vi "Exercise 6.1 PID Host GUI DataLog.vi"() -> ()   [LabVIEW 2014]
doc: "This example demonstrates how to implement a STM client which receives messages from the server.\n\nThe server needs to be started before the client."
uses:
  <vilib>/NI/STM/compatibility/STM Read Meta Data (TCP Ref).vi
  <vilib>/NI/STM/compatibility/STM Read Message (TCP).vi
  <vilib>/Utility/file.llb/Write To Spreadsheet File (DBL).vi
  <vilib>/Utility/file.llb/Write To Spreadsheet File (string).vi
  <vilib>/NI/STM/compatibility/STM Get Connection Reference (TCP).vi
  <vilib>/wsapi/NI_WebServices.lvlib
  <vilib>/Platform/browser.llb/Open URL in Default Browser (string).vi
panel:
  out "Output (MV)":dbl(graph)
  out "HL":bool
  out "LL":bool
  out "Max":dbl
  out "Min":dbl
  out "SP":dbl(knob) scale=0.0..100.0
  out "PV":dbl(knob) scale=0.0..100.0
  out "Monitor Chart":T1(graph)
  in  "Target IP Address":string="192.168.5.1"
  in  "stop":bool
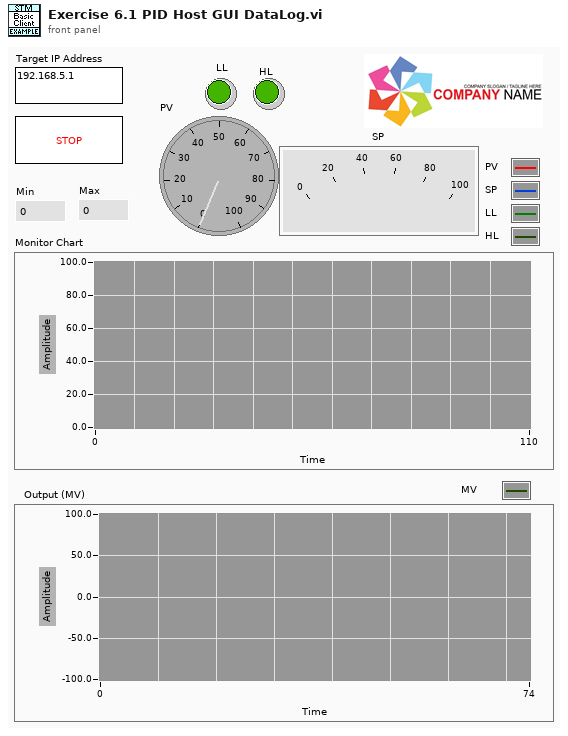
[diagram p1: front panel]
types:
  T1 = cluster{"PV":dbl, "SP":dbl, "Min":dbl, "Max":dbl}
  T2 = typedef "stm_TCP Connection Info.ctl" = cluster{"connection ID":refnum<k5>, "Meta data":T3[]}
  T3 = typedef "stm_MetaDataElement.ctl" = string
  T4 = typedef "imagedata.ctl" = cluster{"image type":i32, "image depth":i32, "image":u8[], "mask":u8[], "colors":u32[], "Rectangle":cluster{"left":i16, "top":i16, "right":i16, "bottom":i16}}
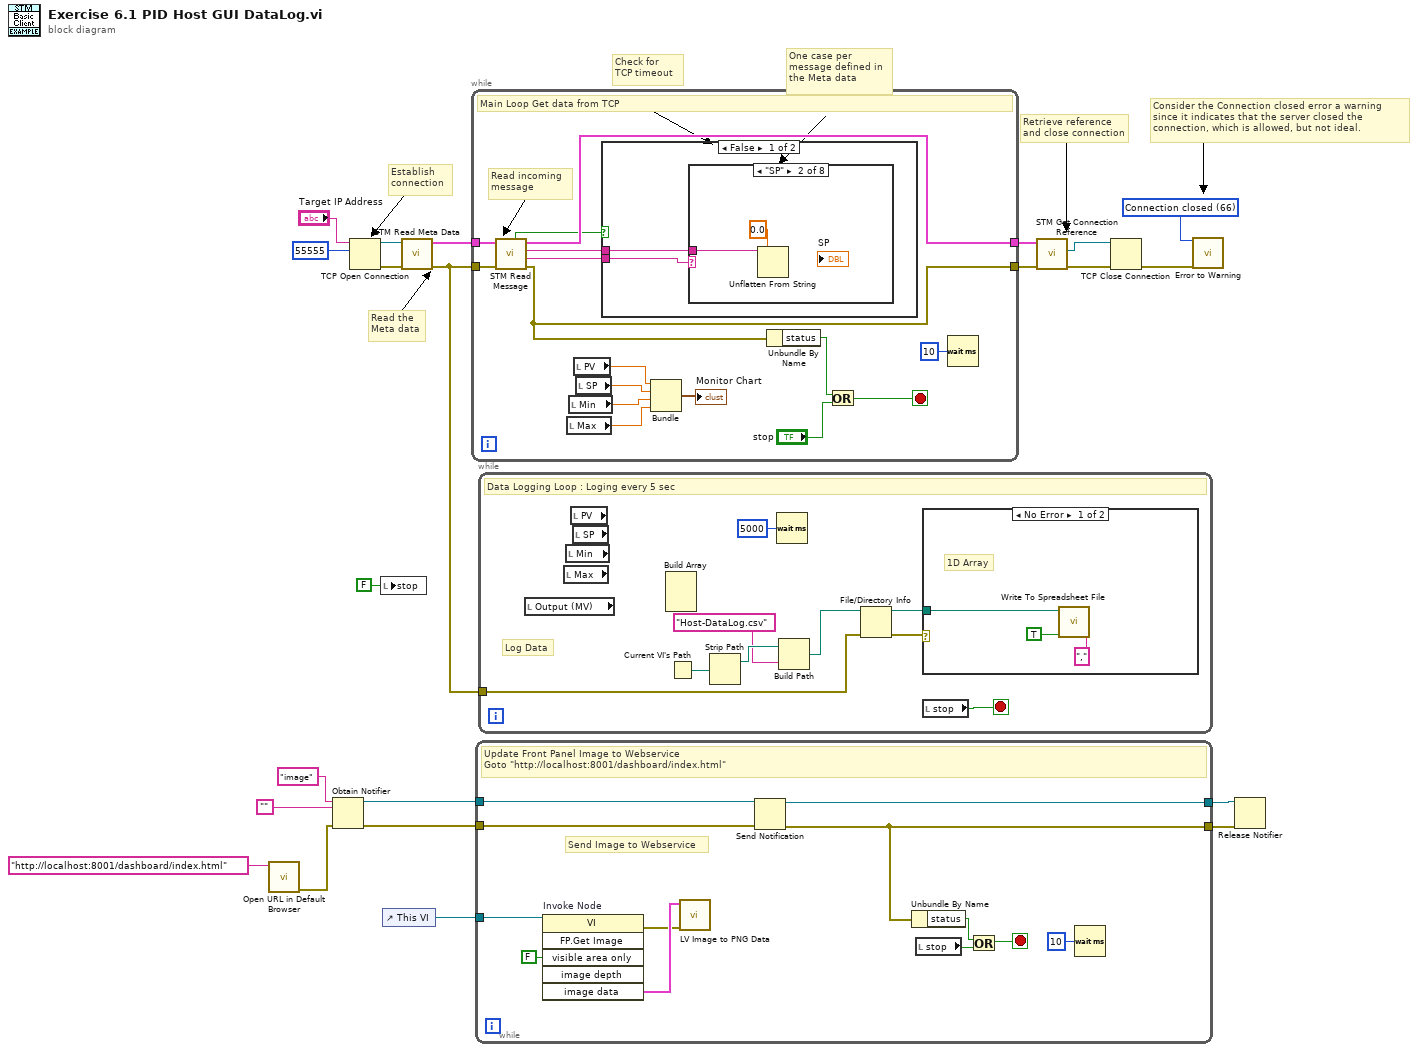
[diagram p0: block diagram]
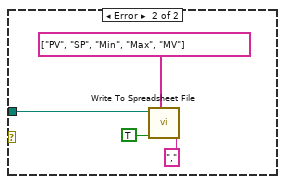
[diagram p2: hidden frame]
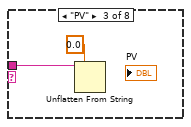
[diagram p4: hidden frame]
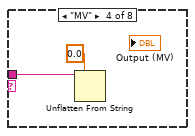
[diagram p5: hidden frame]
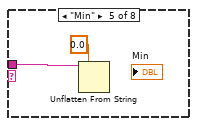
[diagram p6: hidden frame]
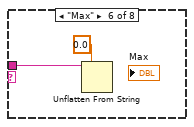
[diagram p7: hidden frame]
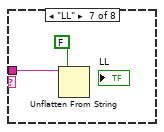
[diagram p8: hidden frame]
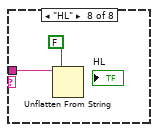
[diagram p9: hidden frame]
diagram:
  w17 = 66 items=["No Error", "Argument Error", "Memory Full", "Out of Zone", "End of File", "File Already Open", "Generic File IO Error", "File Not Found", "File Permission Error", "Disk Full", "Duplicate Path", "Too Many Files Open", "Not Enabled", "Resource File Not Found", "Cannot Add Resource", "Resource Not Found", "Image Not Found", "Image Memory Error", "Pen Does Not Exist", "Config Bad Type", "Config Token Not Found", "Config Parse Error", "Config Memory Error", "Bad External Code Format", "Bad External Code Offset", "External Code Not Present", "Null Window", "Destroy Window Mixup", "Null Menu", "Print Aborted", "Bad Print Record", "Print Driver Error", "Windows Error During Print", "Memory Error During Print", "Print Dialog Error", "Generic Print Error", "Invalid Device Refnum", "Device Not Found", "Device Parameter Error", "Device Unit Error", "Can't Open Device", "Device Call Aborted", "Generic Error", "Cancelled By User", "Object ID Too Low", "Object ID Too High", "Object Not In Heap", "Unknown Heap", "Bad DefProc ID", "DefProc Not In Table", "Message Out Of Range", "Null Method", "Unknown Message", "Manager Call Not Supported", "Bad address", "Connection In progress", "Connection timed out", "Connection is already in progress", "Network attribute not supported", "Network error", "Address in use", "System out of memory", "Connection aborted", "Connection refused", "Connection is not connected", "Connection is already connected", "Connection closed", "Initialize error (interapplication manager)", "Bad occurrence", "Wait on unbound occurrence handler", "Occurrence queue overflow", "Bad path", "Semaphore not signaled", "Unrecognized type (interapplication manager)"] ("1st Error to Convert")
  # "Consider the Connection closed error a warning since it indicates that the server closed the connection, which is allowed, but not ideal."
  # "Retrieve reference and close connection"
  # "Check for\nTCP timeout"
  # "One case per\nmessage defined in\nthe Meta data"
  # "Read the \nMeta data"
  # "Establish\nconnection"
  n1 = call-poly <vilib>:"Open URL in Default Browser.vi"("URL"="http://localhost:8001/dashboard/index.html") -> ("error out"=w2:errorcluster)  [unwired: 5 in, 1 out]
  n2 = Obtain Notifier(name (unnamed)="image", notification data type="", error in (no error)=w2) -> (notifier out=w7:refnum<notifier>, error out=w8:errorcluster)  [unwired: 1 in, 1 out]
  n3 = TCP Open Connection(address="Target IP Address", remote port or service name=u16 55555 ("remote port")) -> (connection ID=w22:refnum<k5>, error out=w20:errorcluster)  [unwired: 1 in, 2 out]
  n4 = local write "stop"(FALSE ("stop")) -> ()
  n5 = control-ref of="This VI"() -> (w10:refnum<vi>)
  n6 = call-poly <vilib>:"STM Read Meta Data.vi"("error in"=w20, "connection ID"=w22) -> ("error out"=w1:errorcluster, "Connection Info Out"=w21:T2)  [unwired: 1 in, 7 out]
  n7 = while {
    tunnel: w21 -> [w38]
    tunnel: w1 -> [w37]
    tunnel: [w36] -> w15
    tunnel: [w33] -> w14
    stop <- w30 stop-if-true
    # "Read incoming\nmessage"
    # "Main Loop Get data from TCP"
    n8 = call-poly <vilib>:"STM Read Message.vi"("error in"=w37, "Connection Info"=w38) -> ("error out"=w33:errorcluster, "Name"=w35:T3, "data string"=w34:string, "Connection Info Out"=w36:T2, "Timed Out?"=w29:bool)  [unwired: 1 in, 4 out]
    n9 = local read "Max"() -> (w25:dbl)
    n10 = local read "Min"() -> (w26:dbl)
    n11 = local read "PV"() -> (w28:dbl)
    n12 = local read "SP"() -> (w27:dbl)
    n13 = case shown="False" w29 {
      tunnel: w35 -> [w39 _]
      tunnel: w34 -> [w40 _]
      frame False {
        n14 = case shown="\"SP\"" w39 {
          tunnel: w40 -> [_ w41 w43 w45 w47 w49 w52 w54]
          frame Default {
          }
          frame "SP" {
            n15 = Unflatten From String(type=0.0, binary string=w41) -> ()  [unwired: 1 in, 5 out]
          }
          frame "PV" {
            n16 = Unflatten From String(type=0.0, binary string=w43) -> ()  [unwired: 1 in, 5 out]
          }
          frame "MV" {
            n17 = Unflatten From String(type=0.0, binary string=w45) -> ()  [unwired: 1 in, 5 out]
          }
          frame "Min" {
            n18 = Unflatten From String(type=0.0, binary string=w47) -> ()  [unwired: 1 in, 5 out]
          }
          frame "Max" {
            n19 = Unflatten From String(type=0.0, binary string=w49) -> ()  [unwired: 1 in, 5 out]
          }
          frame "LL" {
            n20 = Unflatten From String(type=FALSE, binary string=w52) -> ()  [unwired: 1 in, 5 out]
          }
          frame "HL" {
            n21 = Unflatten From String(type=FALSE, binary string=w54) -> ()  [unwired: 1 in, 5 out]
          }
        }
      }
      frame True {
      }
    }
    n22 = Bundle("PV"=w28, "SP"=w27, "Min"=w26, "Max"=w25) -> (→"Monitor Chart":T1)  [unwired: 1 in]
    n23 = Unbundle By Name(w33) -> ("status"=w32:bool)
    n24 = Or(x=w32, y="stop") -> (x .or. y?=w30:bool)
    n25 = Wait (ms)(milliseconds to wait=u32 10) -> ()  [unwired: 1 out]
  }
  n26 = while {
    tunnel: w10 -> [w66]
    tunnel: w7 -> [w64]
    tunnel: w8 -> [w63]
    tunnel: [w62] -> w5
    tunnel: [w61] -> w6
    stop <- w55 stop-if-true
    # "Send Image to Webservice"
    # "Update Front Panel Image to Webservice\nGoto \"http://localhost:8001/dashboard/index.html\""
    n27 = invoke on="Invoke Node" class="VI" method="FP.Get Image"(reference=w66, "visible area only"=FALSE ("Visible Area Only")) -> (error out=w59:errorcluster, "image data"=w60:T4)  [unwired: 4 in, 4 out]
    n28 = call <vilib>:"LV Image to PNG Data.vi"("error in (no error)"=w59, "image data"=w60) -> ()  [unwired: 8 in, 2 out]
    n29 = Send Notification(notifier=w64, error in (no error)=w63) -> (notifier out=w62:refnum<notifier>, error out=w61:errorcluster)  [unwired: 1 in]
    n30 = Unbundle By Name(w61) -> ("status"=w56:bool)
    n31 = local read "stop"() -> (w57:bool)
    n32 = Or(x=w56, y=w57) -> (x .or. y?=w55:bool)
    n33 = Wait (ms)(milliseconds to wait=u32 10) -> ()  [unwired: 1 out]
  }
  n34 = while {
    tunnel: w1 -> [w67]
    stop <- w71 stop-if-true
    # "Log Data"
    # "Data Logging Loop : Loging every 5 sec"
    n35 = local read "Output (MV)"() -> ()  [unwired: 1 out]
    n36 = local read "Max"() -> ()  [unwired: 1 out]
    n37 = local read "Min"() -> ()  [unwired: 1 out]
    n38 = local read "PV"() -> ()  [unwired: 1 out]
    n39 = local read "SP"() -> ()  [unwired: 1 out]
    n40 = Build Array "Build Array"() -> ()  [unwired: 5 in, 1 out]
    n41 = Current VI's Path() -> (path=w73:path)
    n42 = Strip Path(path=w73) -> (stripped path=w75:path)  [unwired: 1 out]
    n43 = Wait (ms)(milliseconds to wait=u32 5000) -> ()  [unwired: 1 out]
    n44 = Build Path(base path=w75, name or relative path="Host-DataLog.csv") -> (appended path=w68:path)
    n45 = File/Directory Info(path=w68, error in=w67) -> (path out=w70:path, error out=w69:errorcluster)  [unwired: 5 out]
    n46 = case shown="No Error" w69 {
      tunnel: w70 -> [w76 w80]
      frame No Error {
        # "1D Array"
        n47 = call-poly <vilib>:"Write To Spreadsheet File.vi"("delimiter (\\t)"="," ("delimiter (\\t)"), "append to file? (new file:F)"=TRUE, "file path (dialog if empty)"=w76) -> ()  [unwired: 5 in, 1 out]
      }
      frame Error {
        n48 = call-poly <vilib>:"Write To Spreadsheet File.vi"("delimiter (\\t)"="," ("delimiter (\\t)"), "append to file? (new file:F)"=TRUE, "1D data"=string[] ["PV", "SP", "Min", "Max", "MV"], "file path (dialog if empty)"=w80) -> ()  [unwired: 4 in, 1 out]
      }
    }
    n49 = local read "stop"() -> (w71:bool)
  }
  n50 = call-poly <vilib>:"STM Get Connection Reference.vi"("error in"=w14, "Connection Info"=w15) -> ("error out"=w12:errorcluster, "connection ID out"=w13:refnum<k5>)  [unwired: 8 out]
  n51 = TCP Close Connection(connection ID=w13, error in (no error)=w12) -> (error out=w16:errorcluster)  [unwired: 2 out]
  n52 = call <vilib>:"Error to Warning.vi"("1st Error to Convert"=w17, "error in"=w16) -> ()  [unwired: 3 in, 11 out]
  n53 = Release Notifier(notifier=w5, error in (no error)=w6) -> ()  [unwired: 1 in, 3 out]
